vi "HeapCreate.vi"(4 "error in (no error)":errorcluster, 6 "MaximumSize (4096 bytes)":i32=4096, 7 "InitialSize (1024 bytes)":i32=1024) -> (0 "error out":errorcluster, 3 "hHeap":i32 format="%.0x")   [LabVIEW 2011]
uses:
  KERNEL32.DLL
panel:
  in  "HEAP_GENERATE_EXCEPTIONS":bool
  in  "HEAP_NO_SERIALIZE":bool
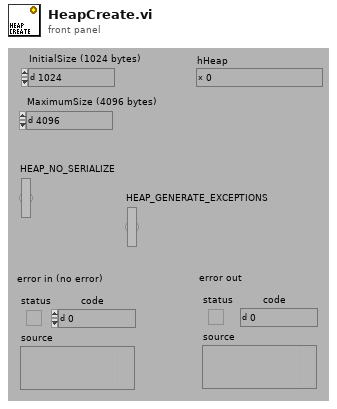
[diagram p1: front panel]
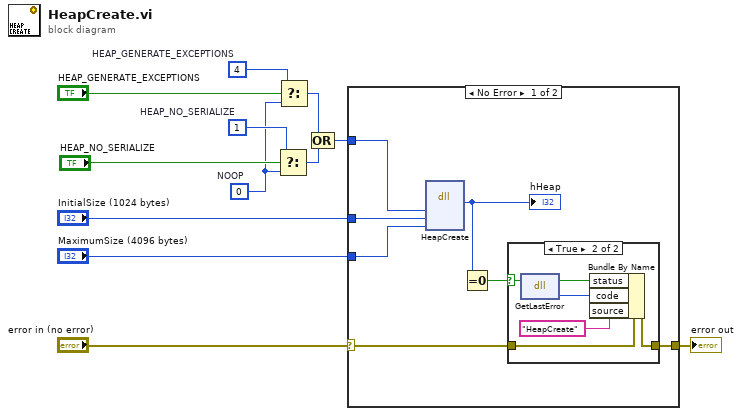
[diagram p0: block diagram]
diagram:
  w1 = u32 0  # NOOP
  w4 = u32 1  # HEAP_NO_SERIALIZE
  w6 = u32 4  # HEAP_GENERATE_EXCEPTIONS
  n1 = Select(t=w4, s="HEAP_NO_SERIALIZE", f=w1) -> (s? t:f=w2:u32)
  n2 = Select(t=w6, s="HEAP_GENERATE_EXCEPTIONS", f=w1) -> (s? t:f=w5:u32)
  n3 = Compound Arithmetic op=OR(w5, w2) -> (w8:u32)
  n4 = case shown="No Error" "error in (no error)" {
    selector: "error in (no error)" -> [w17 w26]
    tunnel: [w16 w26] -> w11
    tunnel: "InitialSize (1024 bytes)" -> [w15 _]
    tunnel: "MaximumSize (4096 bytes)" -> [w14 _]
    tunnel: w8 -> [w13 _]
    frame No Error {
      n5 = dll-call lib="KERNEL32.DLL" fn="HeapCreate" label="HANDLE HeapCreate(\n  DWORD flOptions,       // heap allocation attributes\n  SIZE_T dwInitialSize,  // initial heap size\n  SIZE_T dwMaximumSize   // maximum heap size\n);"("flOptions"=w13, "dwInitialSize"=w15, "dwMaximumSize"=w14) -> ("hHeap"=w19:i32)  [unwired: 6 in, 2 out]
      "hHeap" <- w19
      n6 = Equal To 0?(x=w19) -> (x = 0?=w18:bool)
      n7 = case shown="True" w18 {
        selector: w18 -> [_ w24]
        tunnel: w17 -> [w20 w25]
        tunnel: [w20 w23] -> w16
        frame False {
        }
        frame True {
          n8 = dll-call lib="KERNEL32.DLL" fn="GetLastError"() -> (w22:i32)  [unwired: 3 in, 2 out]
          n9 = Bundle By Name(cluster=w25, "status"=w24, "code"=w22, "source"="HeapCreate") -> (w23:errorcluster)
        }
      }
    }
    frame Error {
    }
  }
  "error out" <- w11
